vi "Send StartLogging.vi"(7 "Message Priority (Normal)":T2=enum."Normal", 8 "error in (no error)":errorcluster, 10 "Mode":T1 items=["Idle", "Snap", "Live", "Capturing", ""], 11 "Message Enqueuer":refnum<class "Message Enqueuer.lvclass">) -> (0 "error out":errorcluster, 3 "Message Enqueuer out":refnum<class "Message Enqueuer.lvclass">)   [LabVIEW 2020, in "DataLogger.lvlib" / "StartLogging Msg.lvclass"]
doc: "This VI sends the message to an actor."
uses:
  StartLogging Msg.lvclass
  <vilib>/ActorFramework/Message Enqueuer/Message Enqueuer.lvclass
  <vilib>/ActorFramework/Message Enqueuer/Message Priority.ctl
  Hardware Layer/Real Hardware/Camera_Prime95B/Camera_Prime95B/Controls/Camera Status.ctl
  C:/Program Files/National Instruments/LabVIEW 2020/vi.lib/ActorFramework/Message/Message.lvclass
  StartLogging Msg.lvclass/StartLogging Msg.ctl
  <vilib>/ActorFramework/Message Enqueuer/Message Enqueuer.lvclass/Message Enqueuer.ctl
  <vilib>/ActorFramework/Message Priority Queue/Priority Enqueue.vi
  Hardware Layer/Real Hardware/Camera_Prime95B/Camera_Prime95B/Camera_Prime95B.lvclass
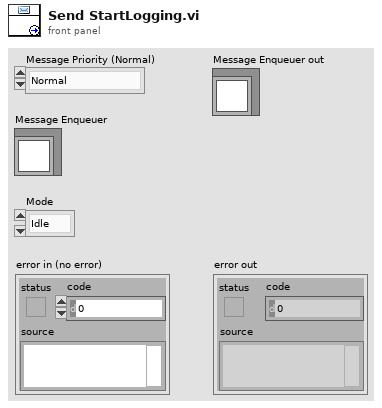
[diagram p1: front panel]
types:
  T1 = typedef "Camera_Prime95B.lvlib/Camera_Prime95B.lvclass/Camera Status.ctl" = i32
  T2 = typedef "Actor Framework.lvlib/Message Enqueuer.lvclass/Message Priority.ctl" = enum16{"Low", "Normal", "High"}
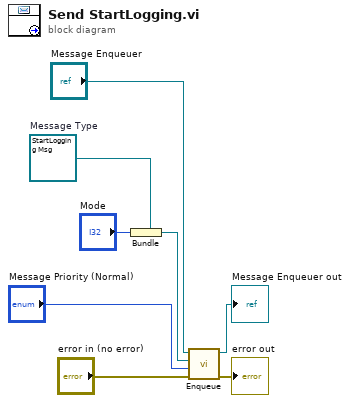
[diagram p0: block diagram]
diagram:
  w2 = refnum<class "StartLogging Msg.lvclass"> refnum  # Message Type
  n1 = Bundle(cluster=w2, "Mode") -> (w3:refnum<class "StartLogging Msg.lvclass">)
  n2 = call <vilib>:"Enqueue.vi"("error in (no error)"="error in (no error)", "Message Priority (Normal)"="Message Priority (Normal)", "Message"=w3, "Message Enqueuer in"="Message Enqueuer") -> ("error out"=→"error out":errorcluster, "Message Enqueuer out"=→"Message Enqueuer out":refnum<class "Message Enqueuer.lvclass">)  [unwired: 6 in]
